vi "circle fit data.vi"(2 "y-offset (b)":dbl, 3 "x-offset (a)":dbl, 4 "radius":dbl, 5 "samples":i32) -> (0 "Y":dbl[](array[numeric]), 1 "X":dbl[](array[numeric]))   [LabVIEW 2023]
doc: "Circle fit data"
uses:
  <vilib>/Analysis/1siggen.llb/Ramp Pattern by Samples.vi
  <vilib>/Analysis/NI_AALBase.lvlib
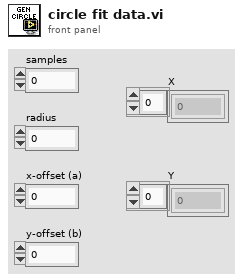
[diagram p1: front panel]
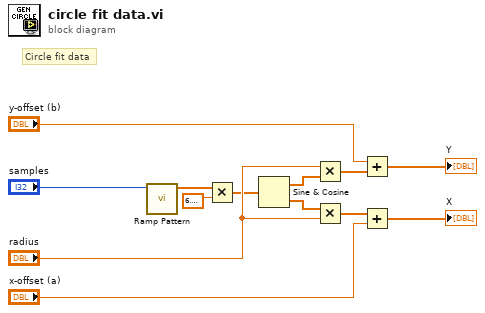
[diagram p0: block diagram]
diagram:
  # "Circle fit data"
  n1 = call-poly <vilib>:"Ramp Pattern.vi"("samples"="samples") -> ("Ramp Pattern"=w3:dbl[])  [unwired: 9 in, 1 out]
  n2 = Multiply(x=w3, y=6.283185307179586) -> (x*y=w5:dbl[])
  n3 = Sine & Cosine(0:w5) -> (1:w8:dbl[], 2:w6:dbl[])
  n4 = Multiply(x="radius", y=w8) -> (x*y=w1:dbl[])
  n5 = Multiply(x=w6, y="radius") -> (x*y=w9:dbl[])
  n6 = Add(x="y-offset (b)", y=w1) -> (x+y=→"Y":dbl[])
  n7 = Add(x=w9, y="x-offset (a)") -> (x+y=→"X":dbl[])
